vi "AutoGenv1.vi"() -> ()   [LabVIEW 2014]
panel:
  in  "Actions":T1(array[cluster])
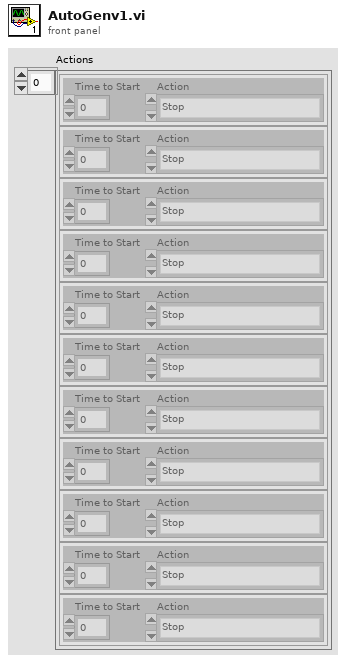
[diagram p1: front panel]
types:
  T1 = cluster{"Time to Start":dbl, "Action":enum16{"Stop", "Drive Forward", "Drive Backwards", "Turn Right", "Turn Left", "Tote Up", "Tote Down", "Doors Open", "Doors Close", "Claw Open", "Claw Close", "Claw Up", "Claw Down", "Claw Stop", "Infeed In", "Infeed Out", "Infeed Off"}}[]
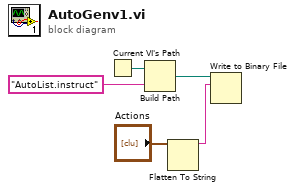
[diagram p0: block diagram]
diagram:
  n1 = Current VI's Path() -> (path=w4:path)
  n2 = Build Path(base path=w4, name or relative path="AutoList.instruct") -> (appended path=w2:path)
  n3 = Flatten To String(anything="Actions") -> (data string=w1:string)  [unwired: 3 in, 2 out]
  n4 = Write to Binary File(file (use dialog)=w2, data=w1) -> ()  [unwired: 4 in, 3 out]
